vi "DigControlSettings.vi"(10 "Digitizer Settings":T1={"Digitizer delay (us) "=0.0, "rf points per line"=2048, "lines per plane"=128, "Samp Rate (Hz)"=100000000.0, "Additional dig delay (us)"=0.0, "Voltage Scale"=0.4, "Pre-Looks"=0, "Offset delay (us)"=0.0, "bits A/D"=8, "Avg Num"=1, "DigTimeOut"=5.0, "Rel Dig Delay"=0.0, "Dig Ch"=0, "LeCroyCluster"={"LeCroy Channels"=[TRUE, FALSE, FALSE, FALSE], "LC read pt offset"=0.0, "Sweep Avg"=FALSE}, "Main Digitizer"=enum."NI Digitizer", "Dig Config"=enum."Single channel", "Digitizer ID Cluster"={"Acqiris/Alazar/SP ID"=[], "NI Instr Handles"=[], "LeCroy VISA"="", "GaGe Handle"={"Handle"=0, "Sample size"=0, "Resolution"=0, "Offset"=0, "Channels"=0, "Boards"=0}, "ATS Ref"="ATS9350", "Acqiris Address"=["PCI::INSTR0"], "ADQRef"=refnum, "adq_cu_ptr"=refnum}, "Trigger Settings"={"Trig Source"=1, "Trig Coupling"=0, "Trig Slope"=0, "Level (mV)"=1500.0}, "Bulk Acq"=FALSE, "Bulk Start Indexes"=[], "Data Ref RF"=refnum, "NI ID/Channel"=[], "Total Dig CH"=5, "Xtra Ann Trig delay (us)"=10.0, "Fix Z Delay?"=FALSE, "One Way Transmission?"=FALSE, "Data Ref Log"=refnum} {"Trigger Settings"."Trig Slope" items=["Positive", "Negative"]; "Trigger Settings"."Level (mV)" format="%.2f"; "Trigger Settings"."Trig Coupling" items=["DC 1 MOhm", "AC 1 MOhm", "DC 50 Ohm", "AC 50 Ohm"]; "Trigger Settings"."Trig Source" items=["Chan 1", "External"]; "Rel Dig Delay" format="%.2f"; "DigTimeOut" format="%.2f"; "Avg Num" min=1; "Offset delay (us)" format="%.2f"; "Additional dig delay (us)" format="%.2f"; "Digitizer delay (us)" format="%.2f"}) -> (1 "Trig Coupling Disable":i32[](array[numeric]), 2 "Ch Coupling Disable":i32[](array[numeric]), 3 "Sampling Rates":T5, 4 "Voltage Scale":T5, 5 "Time Scale/Div":T5)   [LabVIEW 2022 SP3]
uses:
  <vilib>/Utility/miscctls.llb/LVStringsAndValuesArrayTypeDef_DBL.ctl
  DigitizerSettings.ctl
  Digitizer.ctl
  DigConfig.ctl
  DigitizerID.ctl
  C:/Windows/System32/ADQAPI_dotNet_helper.dll
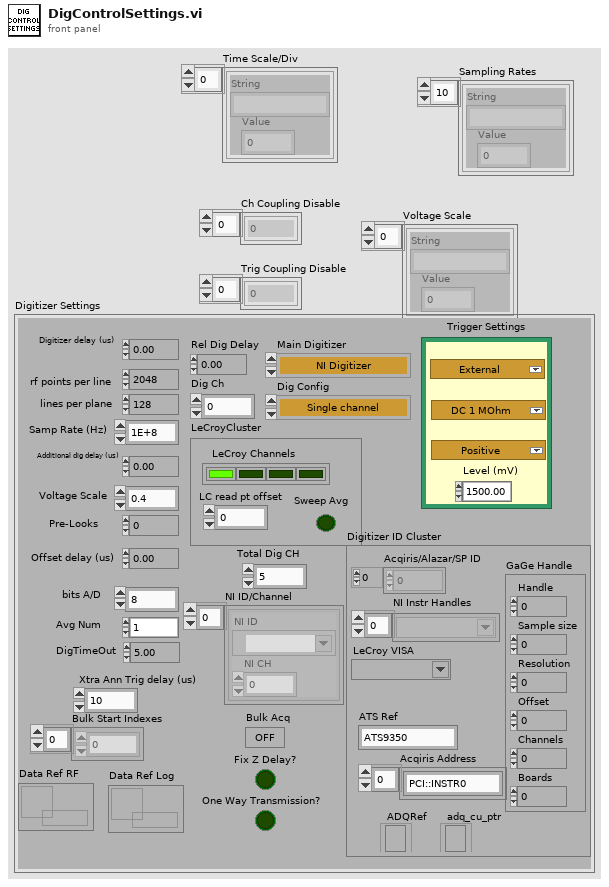
[diagram p1: front panel]
types:
  T1 = typedef "DigitizerSettings.ctl" = cluster{"Digitizer delay (us) ":dbl, "rf points per line":i32, "lines per plane":i32, "Samp Rate (Hz)":dbl, "Additional dig delay (us)":dbl, "Voltage Scale":dbl, "Pre-Looks":i32, "Offset delay (us)":dbl, "bits A/D":i8, "Avg Num":i32, "DigTimeOut":sgl, "Rel Dig Delay":sgl, "Dig Ch":i32, "LeCroyCluster":cluster{"LeCroy Channels":bool[], "LC read pt offset":dbl, "Sweep Avg":bool}, "Main Digitizer":T2, "Dig Config":T3, "Digitizer ID Cluster":T4, "Trigger Settings":cluster{"Trig Source":u16, "Trig Coupling":u16, "Trig Slope":u16, "Level (mV)":dbl}, "Bulk Acq":bool, "Bulk Start Indexes":i32[], "Data Ref RF":refnum<data-value>, "NI ID/Channel":cluster{"NI ID":refnum<k15>, "NI CH":i32}[], "Total Dig CH":i32, "Xtra Ann Trig delay (us)":dbl, "Fix Z Delay?":bool, "One Way Transmission?":bool, "Data Ref Log":refnum<data-value>}
  T2 = typedef "Digitizer.ctl" = enum16{"Acqiris Digitizer", "NI Digitizer", "LeCroy", "GaGe", "AlazarTech", "No Digitizer", "Teledyne"}
  T3 = typedef "DigConfig.ctl" = enum16{"Single channel", "2 Chans w/ 2 Acqiris", "2 Chans w/ 1 Acqiris", "5-CH Pulser New", "5-CH pulser w/ ann array", "5-pass style ann array", "Empty"}
  T4 = typedef "DigitizerID.ctl" = cluster{"Acqiris/Alazar/SP ID":u32[], "NI Instr Handles":refnum<k15>[], "LeCroy VISA":refnum<visa-resource-name>, "GaGe Handle":cluster{"Handle":u32, "Sample size":u32, "Resolution":i32, "Offset":i32, "Channels":u32, "Boards":u32}, "ATS Ref":string, "Acqiris Address":string[], "ADQRef":refnum<k24>, "adq_cu_ptr":refnum<k24>}
  T5 = typedef "LVStringsAndValuesArrayTypeDef_DBL.ctl" = cluster{"String":string, "Value":dbl}[]
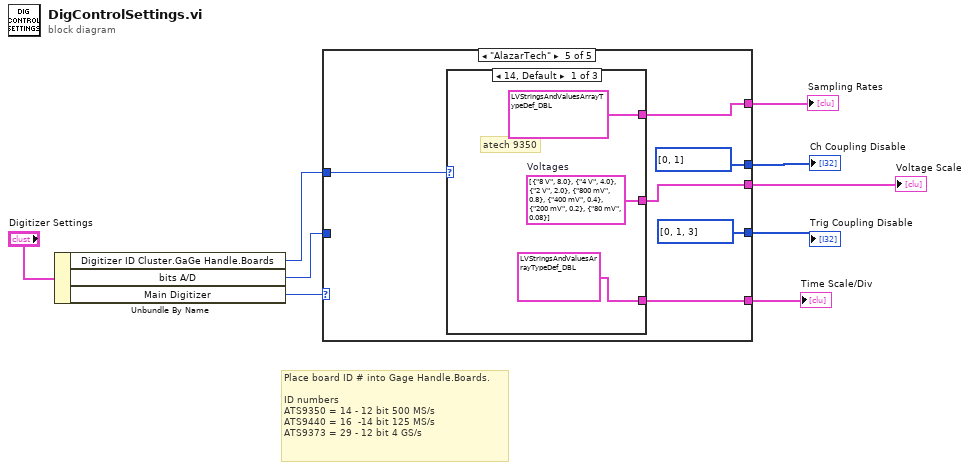
[diagram p0: block diagram]
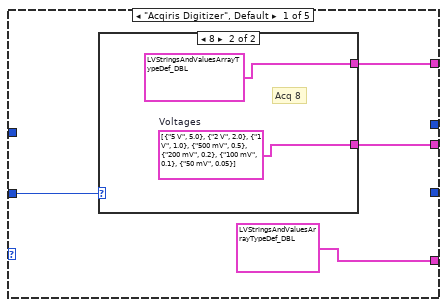
[diagram p2: hidden frame]
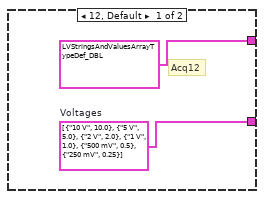
[diagram p3: hidden frame]
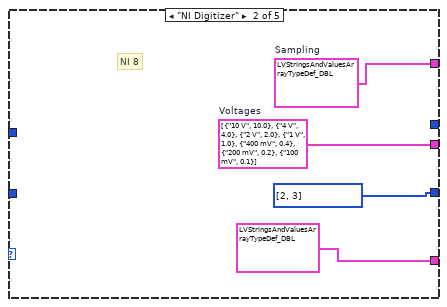
[diagram p4: hidden frame]
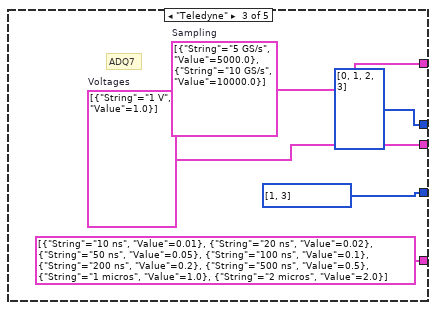
[diagram p5: hidden frame]
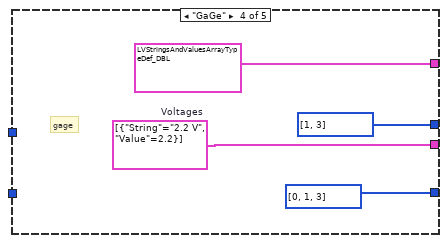
[diagram p6: hidden frame]
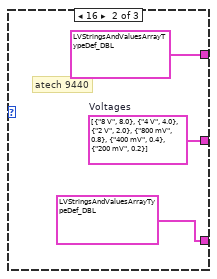
[diagram p7: hidden frame]
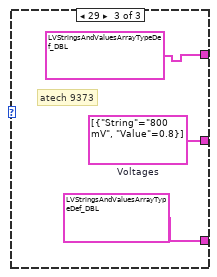
[diagram p8: hidden frame]
diagram:
  # "Place board ID # into Gage Handle.Boards.\n\nID numbers\nATS9350 = 14 - 12 bit 500 MS/s\nATS9440 = 16  -14 bit 125 MS/s\nATS9373 = 29 - 12 bit 4 GS/s"
  n1 = Unbundle By Name("Digitizer Settings") -> ("Digitizer ID Cluster.GaGe Handle.Boards"=w1:u32, "bits A/D"=w2:i8, "Main Digitizer"=w3:T2)
  n2 = case shown="\"AlazarTech\"" w3 {
    tunnel: [_ _ i32[] [0, 1, 2, 3] ("Disabled Items []") i32[] [1, 3] ("Disabled Items []") i32[] [0, 1] ("Disabled Items []")] -> w5
    tunnel: [_ i32[] [2, 3] ("Disabled Items []") i32[] [1, 3] ("Disabled Items []") i32[] [0, 1, 3] ("Disabled Items []") i32[] [0, 1, 3] ("Disabled Items []")] -> w6
    tunnel: [T5 [{"String"="100 ns", "Value"=0.1}, {"String"="200 ns", "Value"=0.2}, {"String"="500 ns", "Value"=0.5}, {"String"="1 micros", "Value"=1.0}, {"String"="2 micros", "Value"=2.0}, {"String"="5 micros", "Value"=5.0}, {"String"="10 micros", "Value"=10.0}, {"String"="20 micros", "Value"=20.0}, {"String"="50 micros", "Value"=50.0}, {"String"="100 micros", "Value"=100.0}, {"String"="200 micros", "Value"=200.0}, {"String"="500 micros", "Value"=500.0}, {"String"="1 ms", "Value"=1000.0}, {"String"="2 ms", "Value"=2000.0}, {"String"="5 ms", "Value"=5000.0}, {"String"="10 ms", "Value"=10000.0}, {"String"="20 ms", "Value"=20000.0}, {"String"="50 ms", "Value"=50000.0}, {"String"="100 ms", "Value"=100000.0}, {"String"="200 ms", "Value"=200000.0}] ("Strings And Values []") T5 [{"String"="100 ns", "Value"=0.1}, {"String"="200 ns", "Value"=0.2}, {"String"="500 ns", "Value"=0.5}, {"String"="1 micros", "Value"=1.0}, {"String"="2 micros", "Value"=2.0}, {"String"="5 micros", "Value"=5.0}, {"String"="10 micros", "Value"=10.0}, {"String"="20 micros", "Value"=20.0}, {"String"="50 micros", "Value"=50.0}, {"String"="100 micros", "Value"=100.0}, {"String"="200 micros", "Value"=200.0}, {"String"="500 micros", "Value"=500.0}, {"String"="1 ms", "Value"=1000.0}, {"String"="2 ms", "Value"=2000.0}, {"String"="5 ms", "Value"=5000.0}, {"String"="10 ms", "Value"=10000.0}, {"String"="20 ms", "Value"=20000.0}, {"String"="50 ms", "Value"=50000.0}, {"String"="100 ms", "Value"=100000.0}, {"String"="200 ms", "Value"=200000.0}] ("Strings And Values []") T5 [{"String"="10 ns", "Value"=0.01}, {"String"="20 ns", "Value"=0.02}, {"String"="50 ns", "Value"=0.05}, {"String"="100 ns", "Value"=0.1}, {"String"="200 ns", "Value"=0.2}, {"String"="500 ns", "Value"=0.5}, {"String"="1 micros", "Value"=1.0}, {"String"="2 micros", "Value"=2.0}] ("Strings And Values []") _ w32] -> w7
    tunnel: [w12 w19 w25 T5 [{"String"="1 MS/s", "Value"=1.0}, {"String"="2 MS/s", "Value"=2.0}, {"String"="5 MS/s\n", "Value"=5.0}, {"String"="10 MS/s", "Value"=10.0}, {"String"="25 MS/s", "Value"=25.0}, {"String"="50 MS/s", "Value"=50.0}, {"String"="100 MS/s", "Value"=100.0}, {"String"="200 MS/s", "Value"=200.0}, {"String"="550 MS/s", "Value"=550.0}, {"String"="1.1 GS/s", "Value"=1100.0}] ("Strings And Values []") w34] -> w8
    tunnel: [w11 w18 w24 w27 w33] -> w9
    tunnel: w2 -> [w10 _ _ _ _]
    tunnel: w1 -> [_ _ _ _ w31]
    frame "Acqiris Digitizer", Default {
      n3 = case shown="8" w10 {
        tunnel: [T5 [{"String"="10 MS/s", "Value"=10.0}, {"String"="20 MS/s", "Value"=20.0}, {"String"="25 MS/s\n", "Value"=25.0}, {"String"="40 MS/s", "Value"=40.0}, {"String"="50 MS/s", "Value"=50.0}, {"String"="100 MS/s", "Value"=100.0}, {"String"="200 MS/s", "Value"=200.0}, {"String"="250 MS/s", "Value"=250.0}, {"String"="400 MS/s", "Value"=400.0}] ("Strings And Values []") T5 [{"String"="10 MS/s", "Value"=10.0}, {"String"="20 MS/s", "Value"=20.0}, {"String"="25 MS/s\n", "Value"=25.0}, {"String"="40 MS/s", "Value"=40.0}, {"String"="50 MS/s", "Value"=50.0}, {"String"="100 MS/s", "Value"=100.0}, {"String"="200 MS/s", "Value"=200.0}, {"String"="250 MS/s", "Value"=250.0}, {"String"="400 MS/s", "Value"=400.0}, {"String"="500 MS/s", "Value"=500.0}, {"String"="1 GS/s", "Value"=1000.0}, {"String"="2 GS/s", "Value"=2000.0}] ("Strings And Values []")] -> w12
        tunnel: [w15 w16] -> w11
        frame 12, Default {
          w15 = T5 [{"String"="10 V", "Value"=10.0}, {"String"="5 V", "Value"=5.0}, {"String"="2 V", "Value"=2.0}, {"String"="1 V", "Value"=1.0}, {"String"="500 mV", "Value"=0.5}, {"String"="250 mV", "Value"=0.25}]  # Voltages
          # "Acq12"
        }
        frame 8 {
          w16 = T5 [{"String"="5 V", "Value"=5.0}, {"String"="2 V", "Value"=2.0}, {"String"="1 V", "Value"=1.0}, {"String"="500 mV", "Value"=0.5}, {"String"="200 mV", "Value"=0.2}, {"String"="100 mV", "Value"=0.1}, {"String"="50 mV", "Value"=0.05}]  # Voltages
          # "Acq 8"
        }
      }
    }
    frame "NI Digitizer" {
      w18 = T5 [{"String"="10 V", "Value"=10.0}, {"String"="4 V", "Value"=4.0}, {"String"="2 V", "Value"=2.0}, {"String"="1 V", "Value"=1.0}, {"String"="400 mV", "Value"=0.4}, {"String"="200 mV", "Value"=0.2}, {"String"="100 mV", "Value"=0.1}]  # Voltages
      w19 = T5 [{"String"="10 MS/s", "Value"=10.0}, {"String"="20 MS/s", "Value"=20.0}, {"String"="25 MS/s\n", "Value"=25.0}, {"String"="50 MS/s", "Value"=50.0}, {"String"="100 MS/s", "Value"=100.0}, {"String"="200 MS/s", "Value"=200.0}, {"String"="250 MS/s", "Value"=250.0}, {"String"="500 MS/s", "Value"=500.0}, {"String"="1 GS/s", "Value"=1000.0}]  # Sampling
      # "NI 8"
    }
    frame "Teledyne" {
      w24 = T5 [{"String"="1 V", "Value"=1.0}]  # Voltages
      w25 = T5 [{"String"="5 GS/s", "Value"=5000.0}, {"String"="10 GS/s", "Value"=10000.0}]  # Sampling
      # "ADQ7"
    }
    frame "GaGe" {
      w27 = T5 [{"String"="2.2 V", "Value"=2.2}]  # Voltages
      # "gage"
    }
    frame "AlazarTech" {
      n4 = case shown="14, Default" w31 {
        tunnel: [T5 [{"String"="1 MS/s", "Value"=1.0}, {"String"="2 MS/s", "Value"=2.0}, {"String"="5 MS/s", "Value"=5.0}, {"String"="10 MS/s", "Value"=10.0}, {"String"="20 MS/s", "Value"=20.0}, {"String"="50 MS/s\n", "Value"=50.0}, {"String"="100 MS/s", "Value"=100.0}, {"String"="250 MS/s", "Value"=250.0}, {"String"="500 MS/s", "Value"=500.0}] ("Strings And Values []") T5 [{"String"="1 MS/s", "Value"=1.0}, {"String"="2 MS/s", "Value"=2.0}, {"String"="5 MS/s", "Value"=5.0}, {"String"="10 MS/s", "Value"=10.0}, {"String"="20 MS/s", "Value"=20.0}, {"String"="50 MS/s\n", "Value"=50.0}, {"String"="100 MS/s", "Value"=100.0}, {"String"="125 MS/s", "Value"=125.0}] ("Strings And Values []") T5 [{"String"="1 MS/s", "Value"=1.0}, {"String"="2 MS/s", "Value"=2.0}, {"String"="5 MS/s", "Value"=5.0}, {"String"="10 MS/s", "Value"=10.0}, {"String"="20 MS/s", "Value"=20.0}, {"String"="50 MS/s\n", "Value"=50.0}, {"String"="100 MS/s", "Value"=100.0}, {"String"="200 MS/s", "Value"=200.0}, {"String"="500 MS/s", "Value"=500.0}, {"String"="800 MS/s", "Value"=800.0}, {"String"="1000 MS/s", "Value"=1000.0}, {"String"="1200 MS/s", "Value"=1200.0}, {"String"="1500 MS/s", "Value"=1500.0}, {"String"="2000 MS/s", "Value"=2000.0}, {"String"="3000 MS/s", "Value"=3000.0}, {"String"="4000 MS/s", "Value"=4000.0}] ("Strings And Values []")] -> w34
        tunnel: [w38 w41 w45] -> w33
        tunnel: [T5 [{"String"="200 ns", "Value"=0.2}, {"String"="400 ns", "Value"=0.4}, {"String"="1 micros", "Value"=1.0}, {"String"="2 micros", "Value"=2.0}, {"String"="5 micros", "Value"=5.0}, {"String"="10 micros", "Value"=10.0}, {"String"="20 micros", "Value"=20.0}, {"String"="50 micros", "Value"=50.0}, {"String"="100 micros", "Value"=100.0}] ("Strings And Values []") T5 [{"String"="1 micros", "Value"=1.0}, {"String"="2 micros", "Value"=2.0}, {"String"="5 micros", "Value"=5.0}, {"String"="10 micros", "Value"=10.0}, {"String"="20 micros", "Value"=20.0}, {"String"="50 micros", "Value"=50.0}, {"String"="100 micros", "Value"=100.0}] ("Strings And Values []") T5 [{"String"="25 ns", "Value"=0.025}, {"String"="50 ns", "Value"=0.05}, {"String"="100 ns", "Value"=0.1}, {"String"="200 ns", "Value"=0.2}, {"String"="1 micros", "Value"=1.0}, {"String"="2 micros", "Value"=2.0}, {"String"="5 micros", "Value"=5.0}, {"String"="10 micros", "Value"=10.0}, {"String"="20 micros", "Value"=20.0}, {"String"="50 micros", "Value"=50.0}, {"String"="100 micros", "Value"=100.0}] ("Strings And Values []")] -> w32
        frame 14, Default {
          w38 = T5 [{"String"="8 V", "Value"=8.0}, {"String"="4 V", "Value"=4.0}, {"String"="2 V", "Value"=2.0}, {"String"="800 mV", "Value"=0.8}, {"String"="400 mV", "Value"=0.4}, {"String"="200 mV", "Value"=0.2}, {"String"="80 mV", "Value"=0.08}]  # Voltages
          # "atech 9350"
        }
        frame 16 {
          w41 = T5 [{"String"="8 V", "Value"=8.0}, {"String"="4 V", "Value"=4.0}, {"String"="2 V", "Value"=2.0}, {"String"="800 mV", "Value"=0.8}, {"String"="400 mV", "Value"=0.4}, {"String"="200 mV", "Value"=0.2}]  # Voltages
          # "atech 9440"
        }
        frame 29 {
          w45 = T5 [{"String"="800 mV", "Value"=0.8}]  # Voltages
          # "atech 9373"
        }
      }
    }
  }
  "Voltage Scale" <- w9
  "Sampling Rates" <- w8
  "Time Scale/Div" <- w7
  "Trig Coupling Disable" <- w6
  "Ch Coupling Disable" <- w5
